vi "Pairwise_Distances_Argmin.vi"(8 "error in":errorcluster caption="entrée d'erreur", 9 "Y":string[][](array[string]), 10 "X":string[][](array[string]), 11 "pairwise_distances_argmin":T2={"axis"=1, "metric "="euclidean", "metric_kwargs"={"metric"=[], "kwargs"=[]}}) -> (0 "error out":errorcluster caption="sortie d'erreur", 3 "Data":T1)   [LabVIEW 2020]
doc: "Compute minimum distances between one point and a set of points.\n\nThis function computes for each row in X, the index of the row of Y which is closest (according to the specified distance).\n\nThis is mostly equivalent to calling:\n\npairwise_distances(X, Y=Y, metric=metric).argmin(axis=axis)\n\nbut uses much less memory, and is faster for large arrays.\n\nThis function works with dense 2D arrays only.\n\nParameters :\n\n- X : array-like\nArrays containing points. Respective shapes (n_samples1, n_features) and (n_samples2, n_features)\n\n- Y : array-like\nArrays containing points. Respective shapes (n_samples1, n_features) and (n_samples2, n_features)\n\n- axis : int, optional, default 1\nAxis along which the argmin and distances are to be computed.\n\n- metric : string or callable\nmetric to use for distance computation. Any metric from scikit-learn or scipy.spatial.distance can be used.\n\nIf metric is a callable function, it is called on each pair of instances (rows) and the resulting value recorded. The callable should take two arrays as input and return one value indicating the distance between them. This works for Scipy’s metrics, but is less efficient than passing the metric name as a string.\n\nDistance matrices are not supported.\n\nValid values for metric are :\n\nfrom scikit-learn: [‘cityblock’, ‘cosine’, ‘euclidean’, ‘l1’, ‘l2’, ‘manhattan’]\n\nfrom scipy.spatial.distance: [‘braycurtis’, ‘canberra’, ‘chebyshev’, ‘correlation’, ‘dice’, ‘hamming’, ‘jaccard’, ‘kulsinski’, ‘mahalanobis’, ‘minkowski’, ‘rogerstanimoto’, ‘russellrao’, ‘seuclidean’, ‘sokalmichener’, ‘sokalsneath’, ‘sqeuclidean’, ‘yule’]\n\n- metric_kwargs : dict\nkeyword arguments to pass to specified metric function.\n\nReturns :\n\n- argmin : numpy.ndarray\nY[argmin[i], :] is the row in Y that is closest to X[i, :]."
uses:
  Argmin.lvclass
panel:
  out "Argmin.lvclass":refnum<class "Argmin.lvclass">
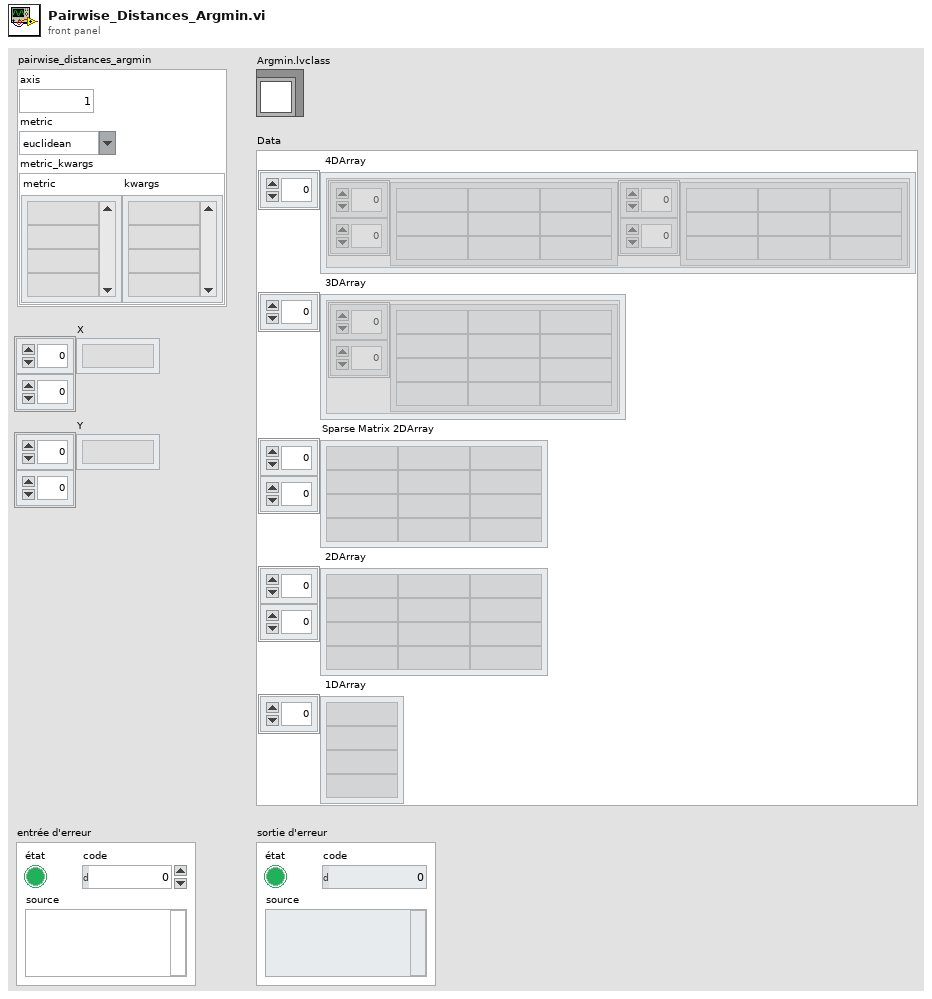
[diagram p1: front panel]
types:
  T1 = cluster{" 4DArray":cluster{"1":string[][], "2":string[][]}[], " 3DArray":cluster{"Tableau":string[][]}[], "Sparse Matrix 2DArray":string[][], " 2DArray":string[][], " 1DArray":string[]}
  T2 = cluster{"axis":i32, "metric ":string, "metric_kwargs":cluster{"metric":string[], "kwargs":string[]}}
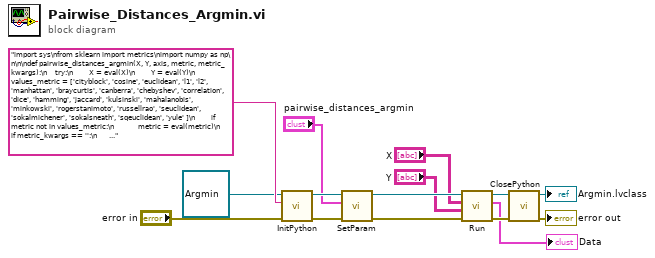
[diagram p0: block diagram]
diagram:
  n1 = call-dynamic "InitPython.vi"("error in (no error)"="error in", "Python Instruction"="import sys\nfrom sklearn import metrics\nimport numpy as np\n\n\ndef pairwise_distances_argmin(X, Y, axis, metric, metric_kwargs):\n    try:\n        X = eval(X)\n        Y = eval(Y)\n        values_metric = ['cityblock', 'cosine', 'euclidean', 'l1', 'l2', 'manhattan', 'braycurtis', 'canberra', 'chebyshev', 'correlation', 'dice', 'hamming', 'jaccard', 'kulsinski', 'mahalanobis', 'minkowski', 'rogerstanimoto', 'russellrao', 'seuclidean', 'sokalmichener', 'sokalsneath', 'sqeuclidean', 'yule' ]\n        if metric not in values_metric:\n            metric = eval(metric)\n        if metric_kwargs == '':\n            metric_kwargs = None\n        else:\n            metric_kwargs= eval(metric_kwargs) \n        pairwise_distances_argmin = metrics.pairwise_distances_argmin(X, Y, axis, metric, metric_kwargs)\n        pairwise_distances_argmin = pairwise_distances_argmin.tolist()\n        return str(pairwise_distances_argmin)\n    except:\n        erreur = sys.exc_info()\n        typerr = u\"%s\" % (erreur[0])\n        typerr = typerr[typerr.find(\"'\")+1:typerr.rfind(\"'\")]\n        msgerr = u\"%s\" % (erreur[1])\n        message = str('/!\\\\ {0} : {1}'. format(typerr,msgerr))\n        return message", "Scikit-learn en entrée"=refnum<class "Argmin.lvclass"> refnum ("Argmin.lvclass")) -> ("error out"=w11:errorcluster, "Scikit-learn en sortie"=w12:refnum<class "Argmin.lvclass">)  [unwired: 7 in]
  n2 = call-dynamic "SetParam.vi"("error in (no error)"=w11, "pairwise_distances_argmin"="pairwise_distances_argmin", "Argmin.lvclass"=w12) -> ("error out"=w9:errorcluster, "Argmin.lvclass"=w8:refnum<class "Argmin.lvclass">)  [unwired: 7 in]
  n3 = call-dynamic "Run.vi"("error in (no error)"=w9, "Y"="Y", "X"="X", "Argmin.lvclass"=w8) -> ("error out"=w6:errorcluster, "Data"=→"Data":T1, "Argmin.lvclass"=w7:refnum<class "Argmin.lvclass">)  [unwired: 5 in]
  n4 = call-dynamic "ClosePython.vi"("error in (no error)"=w6, "Scikit-learn en entrée"=w7) -> ("error out"=→"error out":errorcluster, "Scikit-learn en sortie"=→"Argmin.lvclass":refnum<class "Argmin.lvclass">)  [unwired: 8 in]
